vi "Read Config Version.vi"(8 "error in (no error)":errorcluster, 11 "SequenceNode in":refnum<class "SequenceNode.lvclass">) -> (0 "error out":errorcluster, 2 "Config Version":string, 3 "SequenceNode out":refnum<class "SequenceNode.lvclass">)   [LabVIEW 2015, in "SequenceNode.lvclass"]
uses:
  SequenceNode.lvclass
  SequenceNode.lvclass/SequenceNode.ctl
  Prototype/classes/Sequence/Config/Sequence Config.lvclass
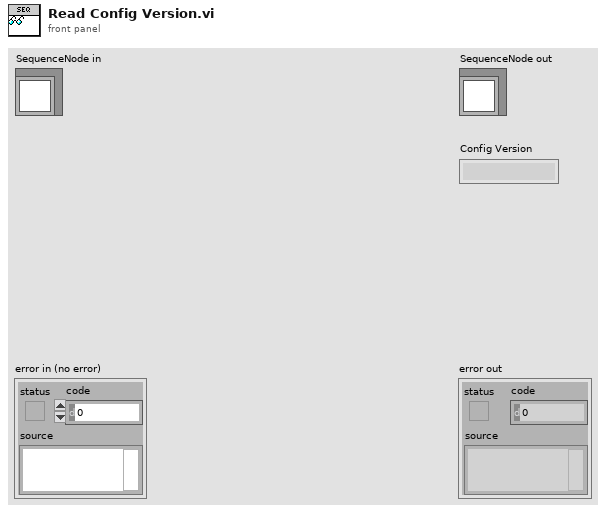
[diagram p1: front panel]
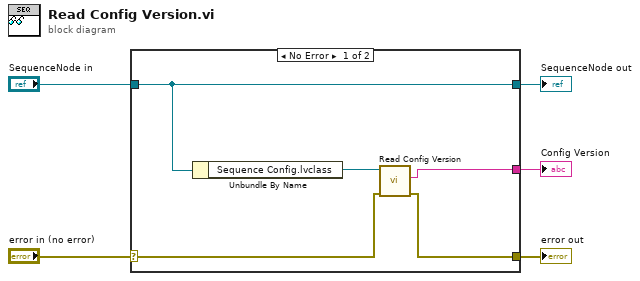
[diagram p0: block diagram]
diagram:
  n1 = case shown="No Error" "error in (no error)" {
    selector: "error in (no error)" -> [w7 w11]
    tunnel: [w6 w11] -> w4
    tunnel: [w10 w12] -> w2
    tunnel: "SequenceNode in" -> [w10 w12]
    tunnel: [w8 _] -> w1
    frame No Error {
      n2 = Unbundle By Name(w10) -> ("Sequence Config.lvclass"=w9:refnum<class "Sequence Config.lvclass">)
      n3 = call-dynamic "Read Config Version.vi"("error in (no error)"=w7, "Sequence Config in"=w9) -> ("error out"=w6:errorcluster, "String"=w8:string)  [unwired: 7 in, 1 out]
    }
    frame Error {
    }
  }
  "error out" <- w4
  "SequenceNode out" <- w2
  "Config Version" <- w1
